vi "process.vi"(8 "error in (no error)":errorcluster, 10 "destination image in (channels)":refnum<class "Image.lvclass">[](array[class]), 11 "DL090216RangeOffsetImageProcessor in":refnum<class "ImageProcessorDL090216RangeOffset.lvclass">) -> (0 "error out":errorcluster, 2 "destination image out (channels)":refnum<class "Image.lvclass">[](array[class]), 3 "DL090216RangeOffsetImageProcessor out":refnum<class "ImageProcessorDL090216RangeOffset.lvclass">)   [LabVIEW 2010, in "ImageProcessorDL090216RangeOffset.lvclass"]
uses:
  ImageProcessorDL090216RangeOffset.lvclass
  common/classes/Image/Image/Image.lvclass
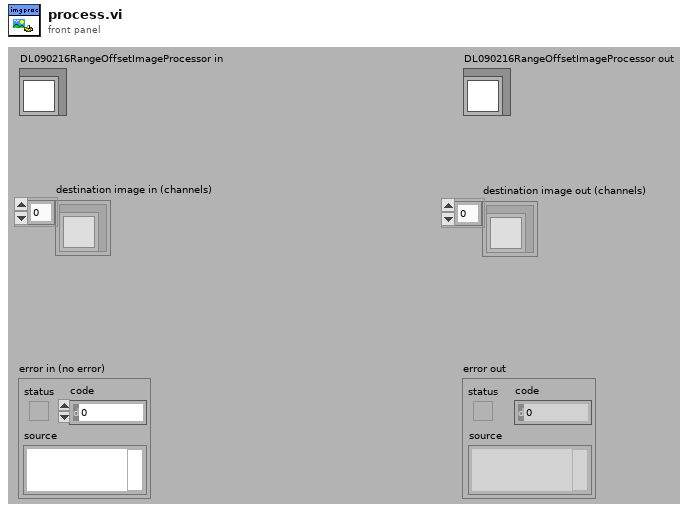
[diagram p1: front panel]
types:
  T1 = typedef "range_offset_cluster.ctl" = cluster{"range":dbl, "offset":dbl}
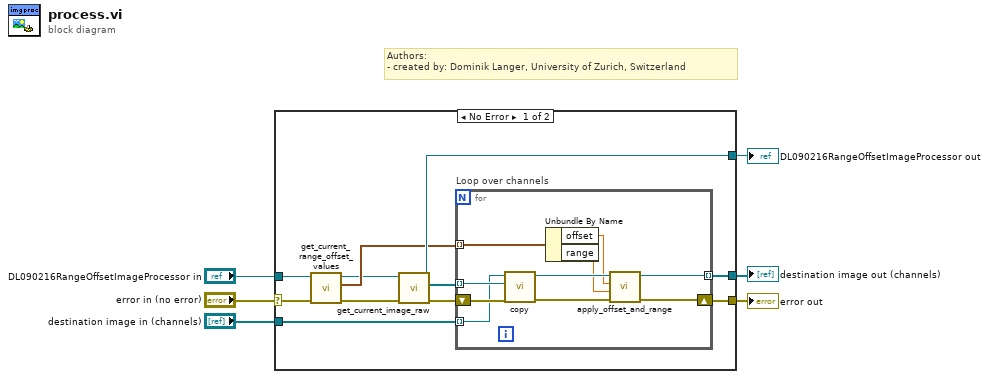
[diagram p0: block diagram]
diagram:
  # "Authors: \n- created by: Dominik Langer, University of Zurich, Switzerland"
  n1 = case shown="No Error" "error in (no error)" {
    selector: "error in (no error)" -> [w12 w29]
    tunnel: [w14 w29] -> w5
    tunnel: [w10 w28] -> w3
    tunnel: "DL090216RangeOffsetImageProcessor in" -> [w7 w28]
    tunnel: [w15 _] -> w2
    tunnel: "destination image in (channels)" -> [w13 _]
    frame No Error {
      n2 = call-dynamic "get_current_range_offset_values.vi"("error in (no error)"=w12, "DL090216RangeOffsetImageProcessor in"=w7) -> ("error out"=w11:errorcluster, "range offset values (channels)"=w9:T1[], "DL090216RangeOffsetImageProcessor out"=w8:refnum<class "ImageProcessorDL090216RangeOffset.lvclass">)  [unwired: 7 out]
      n3 = call-dynamic "get_current_image_raw.vi"("error in (no error)"=w11, "GenericImageProcessor.lvclass in"=w8) -> ("error out"=w17:errorcluster, "current image (channels)"=w16:refnum<class "Image.lvclass">[], "GenericImageProcessor.lvclass out"=w10:refnum<class "ImageProcessorDL090216RangeOffset.lvclass">)  [unwired: 7 out]
      n4 = for "Loop over channels" {
        tunnel: w16 -> [w25] mode=indexing
        shift-right: [w19] -> w14
        shift-left: w17 -> [w26]
        tunnel: [w18] -> w15 mode=indexing
        tunnel: w9 -> [w27] mode=indexing
        tunnel: w13 -> [w22] mode=indexing
        n5 = call "copy.vi"("error in (no error)"=w26, "image to copy (source)"=w25, "Image in (target)"=w22) -> ("error out"=w24:errorcluster, "Image out"=w23:refnum<class "Image.lvclass">)  [unwired: 7 out]
        n6 = Unbundle By Name(w27) -> ("offset"=w21:dbl, "range"=w20:dbl)
        n7 = call-dynamic "apply_offset_and_range.vi"("error in (no error)"=w24, "range"=w20, "offset"=w21, "Image in"=w23) -> ("error out"=w19:errorcluster, "Image out"=w18:refnum<class "Image.lvclass">)  [unwired: 4 in, 2 out]
      }
    }
    frame Error {
    }
  }
  "error out" <- w5
  "DL090216RangeOffsetImageProcessor out" <- w3
  "destination image out (channels)" <- w2
